vi "Builder.Initialize.vi"(8 "error in (no error)":errorcluster, 11 "Builder in":refnum<class "Builder.lvclass">) -> (0 "error out":errorcluster, 3 "Builder out":refnum<class "Builder.lvclass">)   [LabVIEW 2016, in "DSF.Engine.lvlib" / "Builder.lvclass"]
uses:
  Builder.lvclass
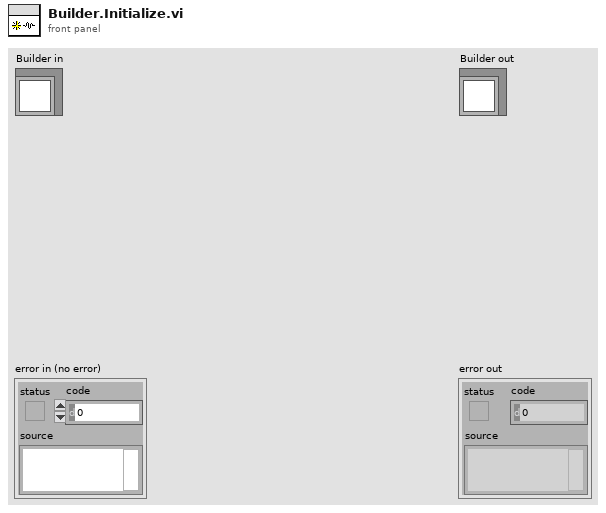
[diagram p1: front panel]
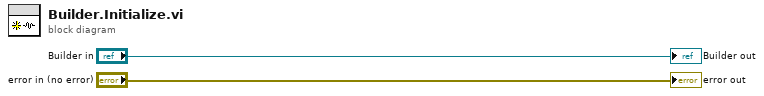
[diagram p0: block diagram]
diagram:
  "error out" <- "error in (no error)"
  "Builder out" <- "Builder in"
